vi "Close.vi"(8 "error in (no error)":errorcluster, 11 "VISA resource name":refnum<visa-resource-name>) -> (0 "error out":errorcluster)   [LabVIEW 2016, in "Agilent 415X Series.lvlib"]
doc: "This VI closes the I/O interface with the instrument."
uses:
  Agilent 415X Series.lvlib
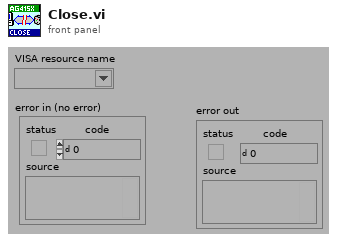
[diagram p1: front panel]
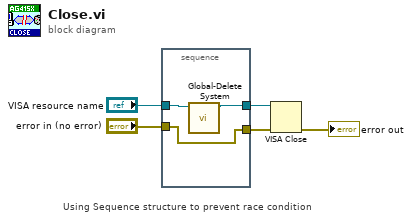
[diagram p0: block diagram]
diagram:
  # "Using Sequence structure to prevent race condition"
  n1 = stacked-sequence {
    tunnel: "VISA resource name" -> [w7]
    tunnel: [w6] -> w3
    tunnel: "error in (no error)" -> [w8]
    tunnel: [w8] -> w1
    frame #0 {
      n2 = call "Global-Delete System.vi"("VISA session"=w7) -> ("VISA resource name out"=w6:refnum<visa-resource-name>)  [unwired: 9 in, 1 out]
    }
  }
  n3 = VISA Close(VISA resource name=w3, error in (no error)=w1) -> (error out=→"error out":errorcluster)
